vi "Configure.vi"(8 "error in (no error)":errorcluster, 11 "DemoDAQ in":refnum<class "DemoDAQ.lvclass">) -> (0 "error out":errorcluster, 3 "DemoDAQ out":refnum<class "DemoDAQ.lvclass">)   [LabVIEW 2020, in "DemoDAQ.lvlib" / "DemoDAQ.lvclass"]
uses:
  DemoDAQ.lvclass
  Hardware Abstraction Layer/Component/DAQ/DAQ/DAQ.lvclass
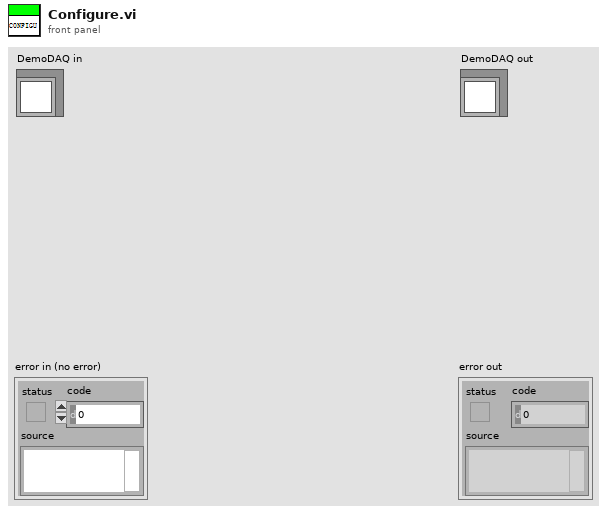
[diagram p1: front panel]
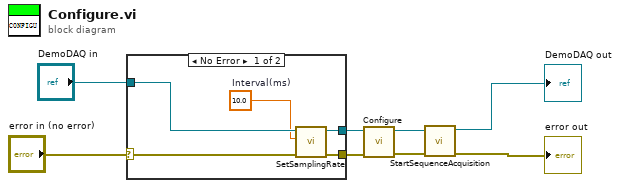
[diagram p0: block diagram]
diagram:
  n1 = case shown="No Error" "error in (no error)" {
    selector: "error in (no error)" -> [w12 w15]
    tunnel: [w11 w15] -> w4
    tunnel: [w9 w14] -> w5
    tunnel: "DemoDAQ in" -> [w13 w14]
    frame No Error {
      w10 = 10.0  # Interval(ms)
      n2 = call-dynamic "SetSamplingRate.vi"("error in (no error)"=w12, "SamplingRate(Hz)"=w10, "Device in"=w13) -> ("error out"=w11:errorcluster, "Device out"=w9:refnum<class "DemoDAQ.lvclass">)  [unwired: 7 in]
    }
    frame Error {
    }
  }
  n3 = call-parent "Configure.vi"("error in (no error)"=w4, "Device in"=w5) -> ("error out"=w8:errorcluster, "Device out"=w2:refnum<class "DemoDAQ.lvclass">)  [unwired: 8 in]
  n4 = call-dynamic "StartSequenceAcquisition.vi"("error in (no error)"=w8, "Device in"=w2) -> ("error out"=→"error out":errorcluster, "Device out"=→"DemoDAQ out":refnum<class "DemoDAQ.lvclass">)  [unwired: 8 in]
